vi "Launch Blower.vi"(7 "Blower":T1, 8 "error in (no error)":errorcluster, 11 "cRIO-CO2 in":refnum<class "cRIO-CO2.lvclass">) -> (0 "error out":errorcluster, 3 "cRIO-CO2 out":refnum<class "cRIO-CO2.lvclass">)   [LabVIEW 2015, in "cRIO-Carbondioxide.lvlib" / "cRIO-CO2.lvlib" / "cRIO-CO2.lvclass"]
uses:
  cRIO-CO2.lvclass
  Blowers Heaters Enumerator.ctl
  <vilib>/ActorFramework/Actor/Actor.lvclass
  cRIO-CO2.lvclass/cRIO-CO2.ctl
  cRIO-CO2 Messages/Log Message Msg/Log Message Msg.lvclass/Log Message Msg.ctl
  <vilib>/ActorFramework/Message Enqueuer/Message Enqueuer.lvclass/Message Enqueuer.ctl
  Freezers Enumerator.ctl
  <vilib>/ActorFramework/Message Enqueuer/Enqueue.vi
  <vilib>/ActorFramework/Message Priority Queue/Priority Enqueue.vi
  <vilib>/ActorFramework/Message Enqueuer/Message Enqueuer.lvclass
  cRIO-CO2 Messages/Log Message Msg/Log Message Msg.lvclass
  Interlocks/Interlock Chain/Interlock Chain.lvclass
  Blower/Blower.lvclass
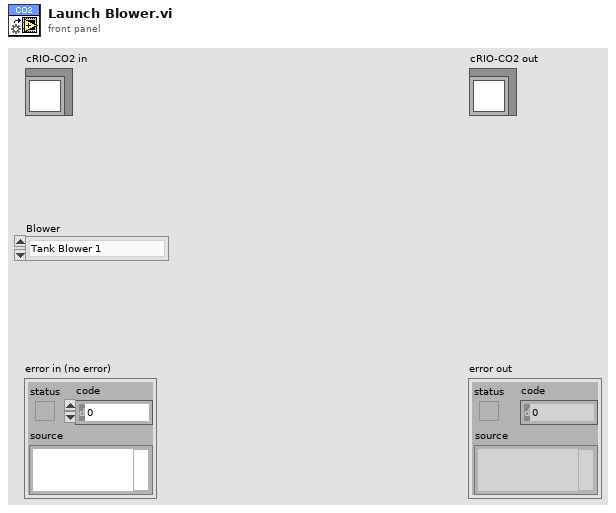
[diagram p1: front panel]
types:
  T1 = typedef "cRIO-Carbondioxide.lvlib/cRIO-CO2.lvlib/cRIO-CO2.lvclass/Blowers Heaters Enumerator.ctl" = enum16{"Tank Blower 1", "Tank Blower 2", "Tank Blower 3", "Tank Blower 4", "Syringe Blower", "Syringe Heater", "Piston Heater", "Undefined"}
  T2 = typedef "cRIO-Carbondioxide.lvlib/cRIO-CO2.lvlib/cRIO-CO2.lvclass/Freezers Enumerator.ctl" = enum16{"Undefined", "Syringe", "Cold Tank 1", "Cold Tank 2", "Cold Tank 3", "Cold Tank 4"}
  T3 = typedef "Dedicated Enqueuers.ctl" = cluster{"Freezers":cluster{"Syringe":refnum<class "Message Enqueuer.lvclass">, "Tank 1":refnum<class "Message Enqueuer.lvclass">, "Tank 2":refnum<class "Message Enqueuer.lvclass">, "Tank 3":refnum<class "Message Enqueuer.lvclass">, "Tank 4":refnum<class "Message Enqueuer.lvclass">}, "Heaters":cluster{"Syringe":refnum<class "Message Enqueuer.lvclass">, "Piston":refnum<class "Message Enqueuer.lvclass">}, "Blowers":cluster{"Tank 1":refnum<class "Message Enqueuer.lvclass">, "Tank 2":refnum<class "Message Enqueuer.lvclass">, "Tank 3":refnum<class "Message Enqueuer.lvclass">, "Tank 4":refnum<class "Message Enqueuer.lvclass">, "Syringe":refnum<class "Message Enqueuer.lvclass">}, "Sample Line":refnum<class "Message Enqueuer.lvclass">, "Storage Line":refnum<class "Message Enqueuer.lvclass">, "Transfer Line":refnum<class "Message Enqueuer.lvclass">, "Syringe Stepper":refnum<class "Message Enqueuer.lvclass">, "Syringe Line":refnum<class "Message Enqueuer.lvclass">, "Capillary Line":refnum<class "Message Enqueuer.lvclass">, "Preparation Line":refnum<class "Message Enqueuer.lvclass">, "Turbo":refnum<class "Message Enqueuer.lvclass">, "Vacuum":refnum<class "Message Enqueuer.lvclass">, "He Line":refnum<class "Message Enqueuer.lvclass">, "Cylinder":refnum<class "Message Enqueuer.lvclass">}
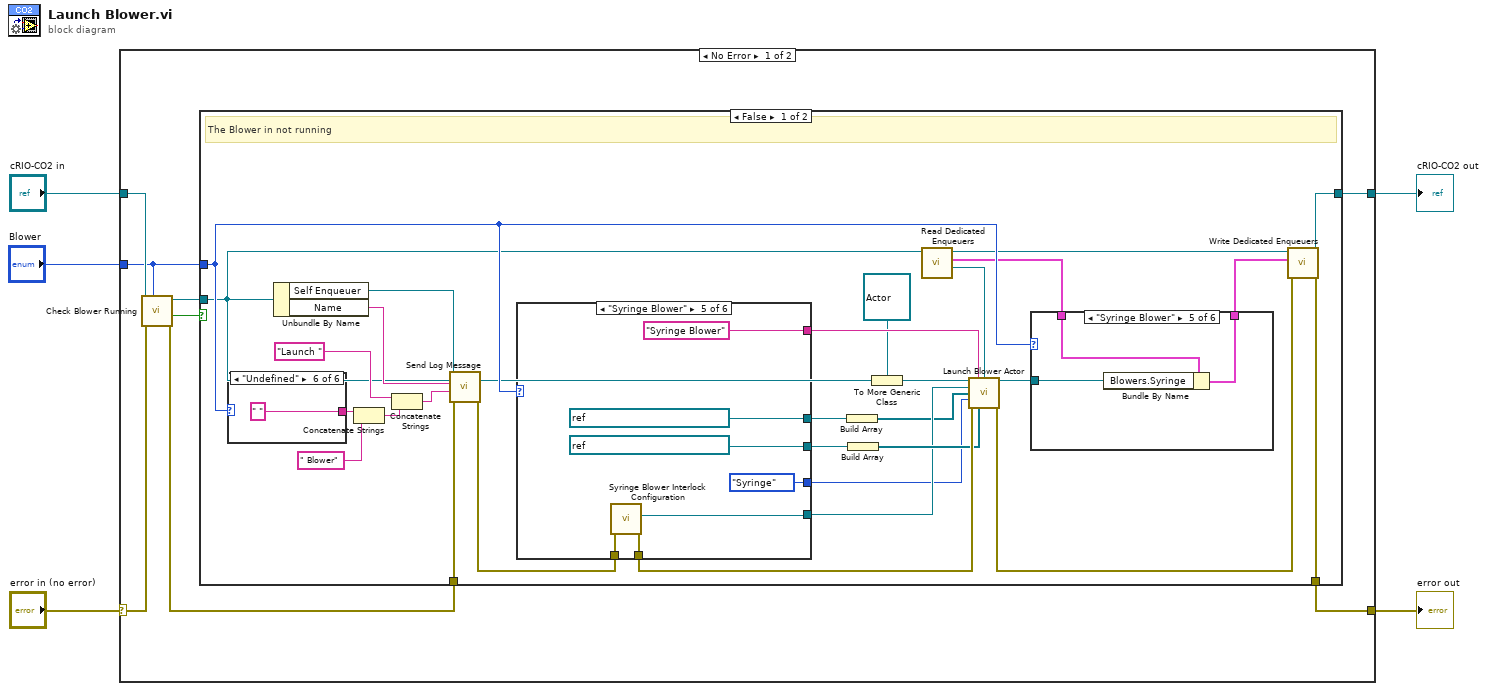
[diagram p0: block diagram]
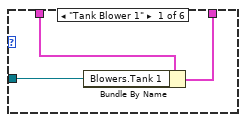
[diagram p2: hidden frame]
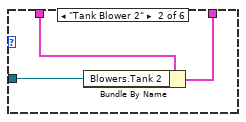
[diagram p3: hidden frame]
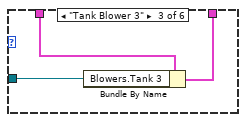
[diagram p4: hidden frame]
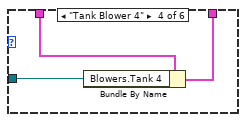
[diagram p5: hidden frame]
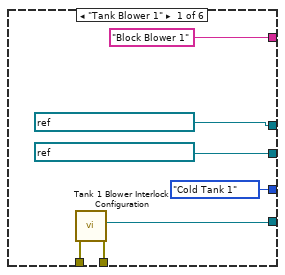
[diagram p7: hidden frame]
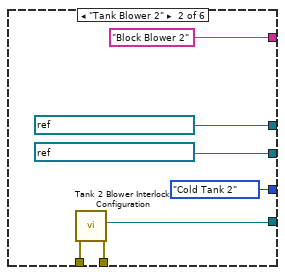
[diagram p8: hidden frame]
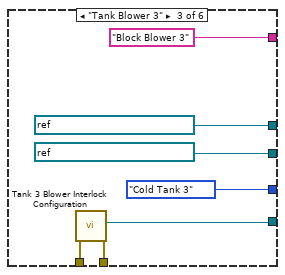
[diagram p9: hidden frame]
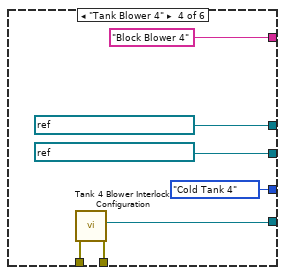
[diagram p10: hidden frame]
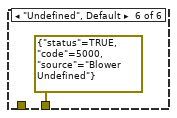
[diagram p11: hidden frame]
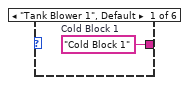
[diagram p12: hidden frame]
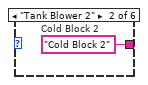
[diagram p13: hidden frame]
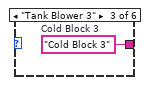
[diagram p14: hidden frame]
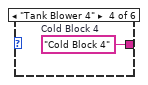
[diagram p15: hidden frame]
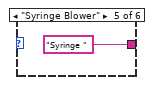
[diagram p16: hidden frame]
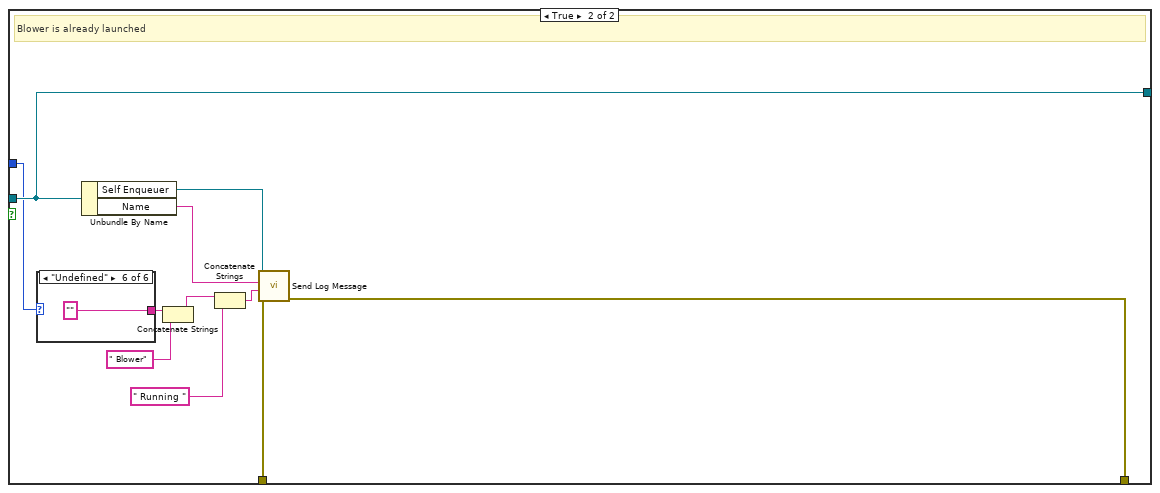
[diagram p17: hidden frame]
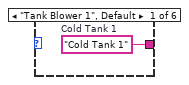
[diagram p18: hidden frame]
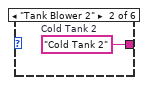
[diagram p19: hidden frame]
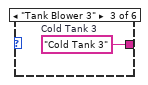
[diagram p20: hidden frame]
diagram:
  n1 = case shown="No Error" "error in (no error)" {
    selector: "error in (no error)" -> [w11 w119]
    tunnel: [w6 w119] -> w4
    tunnel: [w8 w118] -> w2
    tunnel: "cRIO-CO2 in" -> [w13 w118]
    tunnel: "Blower" -> [w12 _]
    frame No Error {
      n2 = call "Check Blower Running.vi"("Blower"=w12, "error in (no error)"=w11, "cRIO-CO2 in"=w13) -> ("error out"=w10:errorcluster, "Running?"=w9:bool, "cRIO-CO2 out"=w7:refnum<class "cRIO-CO2.lvclass">)  [unwired: 6 in]
      n3 = case shown="False" w9 {
        tunnel: w7 -> [w23 w103]
        tunnel: w12 -> [w28 w102]
        tunnel: w10 -> [w34 w107]
        tunnel: [w24 w103] -> w8
        tunnel: [w14 w101] -> w6
        frame False {
          # "The Blower in not running"
          n4 = case shown="\"Undefined\"" w28 {
            tunnel: [w95 w96 w97 w98 "Syringe " " "] -> w41
            frame "Tank Blower 1", Default {
              w95 = "Cold Block 1"  # Cold Block 1
            }
            frame "Tank Blower 2" {
              w96 = "Cold Block 2"  # Cold Block 2
            }
            frame "Tank Blower 3" {
              w97 = "Cold Block 3"  # Cold Block 3
            }
            frame "Tank Blower 4" {
              w98 = "Cold Block 4"  # Cold Block 4
            }
            frame "Syringe Blower" {
            }
            frame "Undefined" {
            }
          }
          n5 = Unbundle By Name(w23) -> ("Self Enqueuer"=w36:refnum<class "Message Enqueuer.lvclass">, "Name"=w42:string)
          n6 = Concatenate Strings(w41, " Blower" ("string")) -> (w39:string)
          n7 = Concatenate Strings("Launch " ("String"), w39) -> (w37:string)
          n8 = call "Send Log Message.vi"("error in (no error)"=w34, "String"=w37, "Source Name"=w42, "Message Enqueuer"=w36) -> ("error out"=w33:errorcluster)  [unwired: 6 in, 1 out]
          n9 = case shown="\"Syringe Blower\"" w28 {
            tunnel: [refnum<k21> "ni.var.psp://10.2.0.20/EtherCAT Master/Device/Mod6 Blowers/Blower1" ("SHV") refnum<k21> "ni.var.psp://10.2.0.20/EtherCAT Master/Device/Mod6 Blowers/Blower2" ("SHV") refnum<k21> "ni.var.psp://10.2.0.20/EtherCAT Master/Device/Mod6 Blowers/Blower3" ("SHV") refnum<k21> "ni.var.psp://10.2.0.20/EtherCAT Master/Device/Mod6 Blowers/Blower4" ("SHV") refnum<k21> "ni.var.io://crio-carbondioxide/EtherCAT Master/Device/Mod6 Blowers/Syringe Blower" ("SHV") _] -> w31
            tunnel: ["Block Blower 1" ("Name") "Block Blower 2" ("Name") "Block Blower 3" ("Name") "Block Blower 4" ("Name") "Syringe Blower" ("Name") _] -> w35
            tunnel: w33 -> [w64 w71 w78 w85 w92 _]
            tunnel: [w63 w70 w77 w84 w91 errorcluster {"status"=TRUE, "code"=5000, "source"="Blower Undefined"} ("error out")] -> w32
            tunnel: [w62 w69 w76 w83 w90 _] -> w20
            tunnel: [refnum<k21> "ni.var.psp://10.2.0.20/AMS Gas SHV/Blowers/Tank Blower 1" ("SHV") refnum<k21> "ni.var.psp://10.2.0.20/AMS Gas SHV/Blowers/Tank Blower 2" ("SHV") refnum<k21> "ni.var.psp://10.2.0.20/AMS Gas SHV/Blowers/Tank Blower 3" ("SHV") refnum<k21> "ni.var.psp://10.2.0.20/AMS Gas SHV/Blowers/Tank Blower 4" ("SHV") refnum<k21> "ni.var.psp://crio-carbondioxide/AMS Gas SHV/Blowers/Syringe Blower" ("SHV") _] -> w19
            tunnel: [Freezers_Enumerator."Cold Tank 1" ("Freezer") Freezers_Enumerator."Cold Tank 2" ("Freezer") Freezers_Enumerator."Cold Tank 3" ("Freezer") Freezers_Enumerator."Cold Tank 4" ("Freezer") Freezers_Enumerator."Syringe" ("Freezer") _] -> w17
            frame "Tank Blower 1" {
              n10 = call "Tank 1 Blower Interlock Configuration.vi"("error in (no error)"=w64) -> ("error out"=w63:errorcluster, "Interlock Chain"=w62:refnum<class "Interlock Chain.lvclass">)  [unwired: 8 in, 1 out]
            }
            frame "Tank Blower 2" {
              n11 = call "Tank 2 Blower Interlock Configuration.vi"("error in (no error)"=w71) -> ("error out"=w70:errorcluster, "Interlock Chain"=w69:refnum<class "Interlock Chain.lvclass">)  [unwired: 8 in, 1 out]
            }
            frame "Tank Blower 3" {
              n12 = call "Tank 3 Blower Interlock Configuration.vi"("error in (no error)"=w78) -> ("error out"=w77:errorcluster, "Interlock Chain"=w76:refnum<class "Interlock Chain.lvclass">)  [unwired: 8 in, 1 out]
            }
            frame "Tank Blower 4" {
              n13 = call "Tank 4 Blower Interlock Configuration.vi"("error in (no error)"=w85) -> ("error out"=w84:errorcluster, "Interlock Chain"=w83:refnum<class "Interlock Chain.lvclass">)  [unwired: 8 in, 1 out]
            }
            frame "Syringe Blower" {
              n14 = call "Syringe Blower Interlock Configuration.vi"("error in (no error)"=w92) -> ("error out"=w91:errorcluster, "Interlock Chain"=w90:refnum<class "Interlock Chain.lvclass">)  [unwired: 8 in, 1 out]
            }
            frame "Undefined", Default {
            }
          }
          n15 = Build Array(w19) -> (w18:refnum<k21>[])
          n16 = Build Array(w31) -> (w29:refnum<k21>[])
          n17 = To More Generic Class(target class=refnum<class "Actor.lvclass"> refnum ("Caller Actor in"), reference=w23) -> (generic class reference=w21:refnum<class "Actor.lvclass">)
          n18 = call "Read Dedicated Enqueuers.vi"("cRIO-CO2 in"=w23) -> ("Qs.DedicatedEnQrs"=w16:refnum<queue>, "Dedicated Enqueuers"=w27:T3, "cRIO-CO2 out"=w26:refnum<class "cRIO-CO2.lvclass">)  [unwired: 7 in, 1 out]
          n19 = call "Launch Blower Actor.vi"("Caller Actor in"=w21, "Name"=w35, "DedicatedEnQrs"=w16, "Interlock Chain"=w20, "SHV Aliases"=w18, "Freezer"=w17, "error in (no error)"=w32, "SHV"=w29) -> ("Caller-To-Actor Enqueuer"=w30:refnum<class "Message Enqueuer.lvclass">, "error out"=w15:errorcluster)  [unwired: 6 in]
          n20 = case shown="\"Syringe Blower\"" w28 {
            tunnel: w27 -> [w45 w48 w51 w54 w57 w58]
            tunnel: w30 -> [w44 w47 w50 w53 w56 _]
            tunnel: [w43 w46 w49 w52 w55 w58] -> w25
            frame "Tank Blower 1" {
              n21 = Bundle By Name(cluster=w45, "Blowers.Tank 1"=w44) -> (w43:T3)
            }
            frame "Tank Blower 2" {
              n22 = Bundle By Name(cluster=w48, "Blowers.Tank 2"=w47) -> (w46:T3)
            }
            frame "Tank Blower 3" {
              n23 = Bundle By Name(cluster=w51, "Blowers.Tank 3"=w50) -> (w49:T3)
            }
            frame "Tank Blower 4" {
              n24 = Bundle By Name(cluster=w54, "Blowers.Tank 4"=w53) -> (w52:T3)
            }
            frame "Syringe Blower" {
              n25 = Bundle By Name(cluster=w57, "Blowers.Syringe"=w56) -> (w55:T3)
            }
            frame "Undefined", Default {
            }
          }
          n26 = call "Write Dedicated Enqueuers.vi"("error in (no error)"=w15, "Dedicated Enqueuers"=w25, "cRIO-CO2 in"=w26) -> ("error out"=w14:errorcluster, "cRIO-CO2 out"=w24:refnum<class "cRIO-CO2.lvclass">)  [unwired: 7 in]
        }
        frame True {
          # "Blower is already launched"
          n27 = case shown="\"Undefined\"" w102 {
            tunnel: [w112 w113 w114 w115 "Syringe " ""] -> w110
            frame "Tank Blower 1", Default {
              w112 = "Cold Tank 1"  # Cold Tank 1
            }
            frame "Tank Blower 2" {
              w113 = "Cold Tank 2"  # Cold Tank 2
            }
            frame "Tank Blower 3" {
              w114 = "Cold Tank 3"  # Cold Tank 3
            }
            frame "Tank Blower 4" {
              w115 = "Cold Tank 4"  # Cold Tank 4
            }
            frame "Syringe Blower" {
            }
            frame "Undefined" {
            }
          }
          n28 = Unbundle By Name(w103) -> ("Self Enqueuer"=w108:refnum<class "Message Enqueuer.lvclass">, "Name"=w111:string)
          n29 = Concatenate Strings(w110, " Blower" ("string")) -> (w106:string)
          n30 = Concatenate Strings(w106, " Running " ("String")) -> (w104:string)
          n31 = call "Send Log Message.vi"("error in (no error)"=w107, "String"=w104, "Source Name"=w111, "Message Enqueuer"=w108) -> ("error out"=w101:errorcluster)  [unwired: 6 in, 1 out]
        }
      }
    }
    frame Error {
    }
  }
  "error out" <- w4
  "cRIO-CO2 out" <- w2
